vi "GetDefaultParams.vi"(8 "error in (no error)":errorcluster, 10 "config file path":path=path "Z:/My Documents/Projects/NistPluggableModules/Scope/ScopePlugins/ScopePluginBaseClass/ScopeBase.ini", 11 "ScopeBase":refnum<class "ScopePluginsBase.lvclass">) -> (0 "error out":errorcluster, 2 "config file path":path=path "Z:/My Documents/Projects/NistPluggableModules/Scope/ScopePlugins/ScopePluginBaseClass/ScopeBase.ini", 3 "ScopeBase":refnum<class "ScopePluginsBase.lvclass">)   [LabVIEW 2018, in "ScopePlugins.lvlib" / "ScopePluginsBase.lvclass"]
uses:
  ScopePluginsBase.lvclass
  C:/Program Files (x86)/National Instruments/LabVIEW 2018/user.lib/NIST/BaseClasses/BasePlugin_class/BasePlugin.lvclass
  Shared/TypeDefs/Acquisition.ctl
  Shared/TypeDefs/Trigger.ctl
  Shared/TypeDefs/Channels.ctl
  Shared/TypeDefs/Channel.ctl
  TypeDefs/InitializeOptions.ctl
  <userlib>/NIST/BaseClasses/BasePlugin_class/BasePlugin.lvclass/BasePlugin.ctl
  ScopePluginsBase.lvclass/ScopePluginsBase.ctl
  <userlib>/NIST/BaseClasses/BasePlugin_class/Accessors/Write PluginIniFilePath.vi
  Accessors/Write Acquisition.vi
  Accessors/Write Trigger.vi
  Accessors/Write Channels.vi
  <userlib>/NIST/BaseClasses/BasePlugin_class/Accessors/Read PluginIniFilePath.vi
  <vilib>/Utility/config.llb/NI_LVConfig.lvlib
  ScopePlugins.lvlib
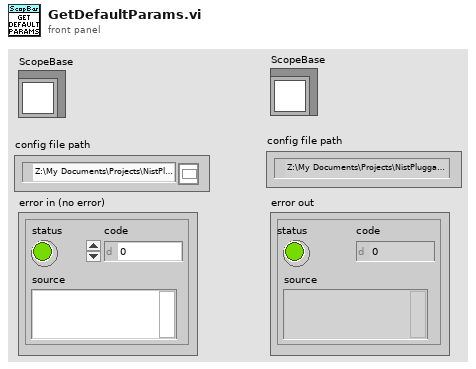
[diagram p1: front panel]
types:
  T1 = typedef "ScopePlugins.lvlib/ScopePluginsBase.lvclass/InitializeOptions.ctl" = cluster{"Reset":bool, "IdQuery":bool, "AutoConfig":bool, "Options String":string, "Synchronize":bool}
  T2 = typedef "ScopePlugins.lvlib/Channels.ctl" = cluster{"Count":i32, "ChannelArray":T3[]}
  T3 = typedef "ScopePlugins.lvlib/Channel.ctl" = cluster{"Enabled":bool, "Name":string, "InputImpedance":dbl, "InputFreqMax":dbl, "ProbeAttn":dbl, "Coupling":enum16{"AC", "DC", "GND"}, "Offset":dbl, "Range":dbl, "Handle":string, "Connected":bool, "Options String ":string}
  T4 = typedef "ScopePlugins.lvlib/Trigger.ctl" = cluster{"Coupling":enum16{"AC", "DC", "LF Reject", "HF Reject", "Noise Reject"}, "Holdoff":dbl, "Level":dbl, "Slope":enum16{"Negative", "Positive"}, "Source":string, "Type":enum16{"Edge", "Width", "Runt", "Glitch", "TV", "Immediate", "AC Line"}}
  T5 = typedef "ScopePlugins.lvlib/Acquisition.ctl" = cluster{"StartTime":dbl, "Type":enum16{"Normal", "PeakDetect", "HighRes", "Envelope", "Average"}, "NumPointsMin":i32, "RecordLength":i32, "SampleRate":dbl, "TimePerRecord":dbl, "SamplingMode ":enum16{"Real Time", "Equivalent Time", "Segment", "Real Time Peak Detect", "Real Time High Resolution", "Peak Detect Segment", "High Resolution Segment"}, "Interpolation":enum16{"No Interpolation", "sin(x)/x", "linear", "1 Point sin(x)/x", "2 Point sin(x)/x", "4 Point sin(x)/x", "8 Point sin(x)/x", "16 Point sin(x)/x"}, "NumAverages":i32, "Resolution":enum16{"Auto", "Bits 9", "Bits 10", "Bits 11", "Bits 12"}, "EnableAveraging":bool, "Continuous":bool}
  T6 = typedef "NI_LVConfig.lvlib/Config Data RefNum.ctl" = refnum<k1>
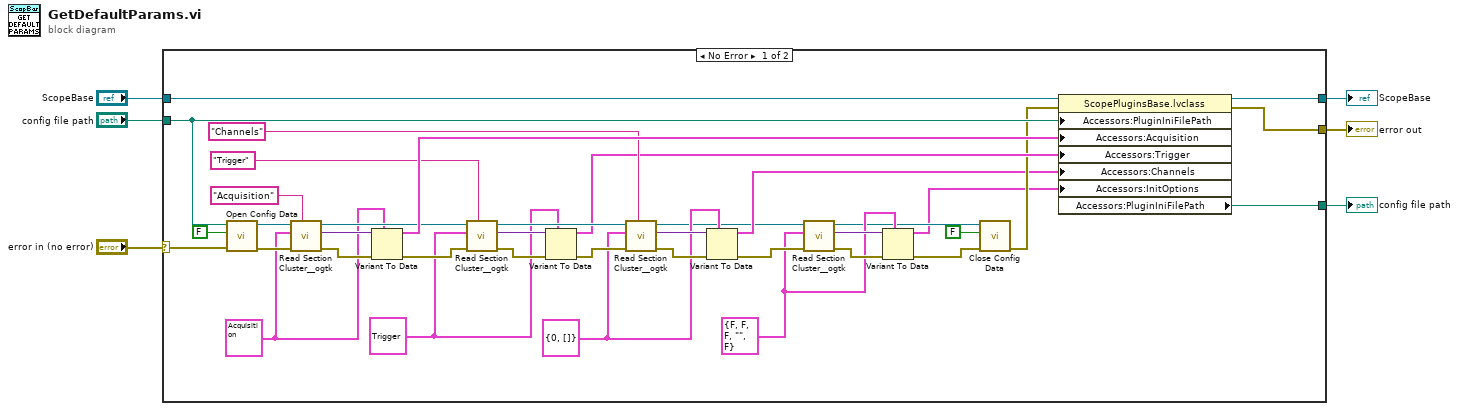
[diagram p0: block diagram]
diagram:
  n1 = case shown="No Error" "error in (no error)" {
    selector: "error in (no error)" -> [w44 w46]
    tunnel: "ScopeBase" -> [w42 w47]
    tunnel: [w41 w47] -> w4
    tunnel: "config file path" -> [w30 w45]
    tunnel: [w18 w45] -> w2
    tunnel: [w21 w46] -> w1
    frame No Error {
      w9 = T1 {"Reset"=FALSE, "IdQuery"=FALSE, "AutoConfig"=FALSE, "Options String"="", "Synchronize"=FALSE} ("InitOptions")
      w13 = T2 {"Count"=0, "ChannelArray"=[]} ("Channels")
      w14 = T4 {"Coupling"=enum."AC", "Holdoff"=0.0, "Level"=0.0, "Slope"=enum."Positive", "Source"="", "Type"=enum."Edge"} ("Trigger")
      w15 = T5 {"StartTime"=0.0, "Type"=enum."Normal", "NumPointsMin"=0, "RecordLength"=0, "SampleRate"=0.0, "TimePerRecord"=0.0, "SamplingMode "=enum."Real Time", "Interpolation"=enum."No Interpolation", "NumAverages"=8, "Resolution"=enum."Auto", "EnableAveraging"=FALSE, "Continuous"=FALSE} ("Acquisition")
      n2 = call <vilib>:"Open Config Data.vi"("error in (no error)"=w44, "create file if necessary (T)"=FALSE, "configuration file path"=w30) -> ("error out"=w22:errorcluster, "refnum"=w23:T6)  [unwired: 6 in, 1 out]
      n3 = call <userlib>:"Read Section Cluster__ogtk.vi"("section (optional)"="Acquisition", "error in (no error)"=w22, "Section Formatted Cluster Type"=w15, "refnum"=w23) -> ("error out"=w38:errorcluster, "Section Formatted Cluster"=w37:variant, "dup refnum"=w34:T6)  [unwired: 3 in, 2 out]
      n4 = Variant To Data(error in=w38, type=w15, Variant=w37) -> (data=w36:T5, error out=w31:errorcluster)
      n5 = call <userlib>:"Read Section Cluster__ogtk.vi"("section (optional)"="Trigger", "error in (no error)"=w31, "Section Formatted Cluster Type"=w14, "refnum"=w34) -> ("error out"=w35:errorcluster, "Section Formatted Cluster"=w33:variant, "dup refnum"=w29:T6)  [unwired: 3 in, 2 out]
      n6 = Variant To Data(error in=w35, type=w14, Variant=w33) -> (data=w24:T4, error out=w28:errorcluster)
      n7 = call <userlib>:"Read Section Cluster__ogtk.vi"("section (optional)"="Channels", "error in (no error)"=w28, "Section Formatted Cluster Type"=w13, "refnum"=w29) -> ("error out"=w27:errorcluster, "Section Formatted Cluster"=w26:variant, "dup refnum"=w11:T6)  [unwired: 3 in, 2 out]
      n8 = Variant To Data(error in=w27, type=w13, Variant=w26) -> (data=w19:T2, error out=w12:errorcluster)
      n9 = call <userlib>:"Read Section Cluster__ogtk.vi"("error in (no error)"=w12, "Section Formatted Cluster Type"=w9, "refnum"=w11) -> ("error out"=w16:errorcluster, "Section Formatted Cluster"=w17:variant, "dup refnum"=w8:T6)  [unwired: 4 in, 2 out]
      n10 = Variant To Data(error in=w16, type=w9, Variant=w17) -> (data=w7:T1, error out=w10:errorcluster)
      n11 = call <vilib>:"Close Config Data.vi"("error in (no error)"=w10, "write file if changed (T)"=FALSE, "refnum"=w8) -> ("error out"=w20:errorcluster)  [unwired: 7 in, 1 out]
      n12 = property class="ScopePluginsBase.lvclass"(reference=w42, error in=w20, "Accessors:PluginIniFilePath"=w30, "Accessors:Acquisition"=w36, "Accessors:Trigger"=w24, "Accessors:Channels"=w19, "Accessors:InitOptions"=w7) -> (reference out=w41:refnum<class "ScopePluginsBase.lvclass">, error out=w21:errorcluster, "Accessors:PluginIniFilePath"=w18:path)
    }
    frame Error {
    }
  }
  "ScopeBase" <- w4
  "error out" <- w1
  "config file path" <- w2
